vi "Configure Accelerometer Range.vi"(8 "error in (no error)":errorcluster, 10 "Range ( 2G )":u16(ring) items=["2G", "6G"], 11 "VISA resource name":refnum<visa-resource-name>) -> (0 "error out":errorcluster, 3 "VISA resource out":refnum<visa-resource-name>)   [LabVIEW 2011, in "Ocean Server OS4000.lvlib"]
doc: "Change Accelerometer maximum measurement range. Options are 2G or 6G\ndefault is 2G output.\n\nImportant Note: 6G output results in less roll and pitch resolution. The 6G range should only be used if the you are trying to measure the effects of X,Y,Z acceleration more than the\nangle of the compass."
uses:
  Ocean Server OS4000.lvlib
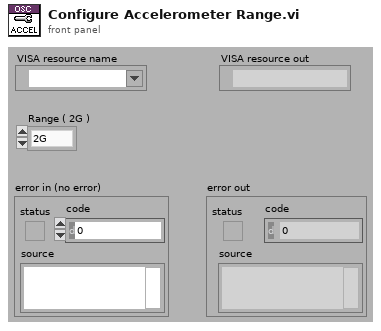
[diagram p1: front panel]
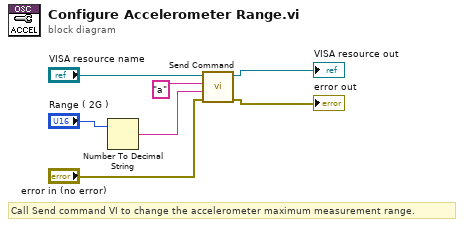
[diagram p0: block diagram]
diagram:
  # "Call Send command VI to change the accelerometer maximum measurement range."
  n1 = Number To Decimal String(number="Range ( 2G )") -> (decimal integer string=w4:string)  [unwired: 1 in]
  n2 = call "Send Command.vi"("error in (no error)"="error in (no error)", "Value"=w4, "Message"="a", "VISA resource name"="VISA resource name") -> ("error out"=→"error out":errorcluster, "VISA resource out"=→"VISA resource out":refnum<visa-resource-name>)  [unwired: 6 in]
